vi "Restarts Monitor (FPGA).vi"() -> ()   [LabVIEW 2019]
uses:
  <vilib>/eio/EIONode/EIONode.xnode
  <vilib>/rvi/eio/common/nirviEmuTemplateMethod_errors.vi
panel:
  in  "Reset":bool
  in  "Loop Timer (uSec)":u32 caption="Count(uSec)"
  out "Actual Pump Starts":u32[](array[numeric])
  in  "Consec Samples":i32
  in  "Threshold (A)":sgl
  out "Currents (A)":sgl[](array[numeric])
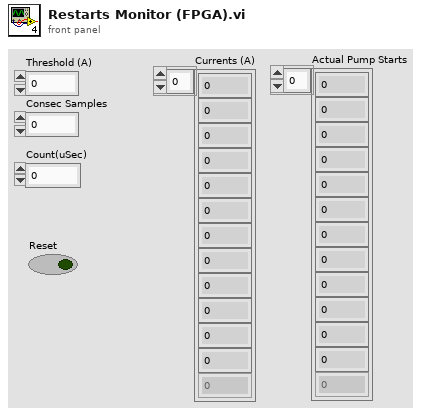
[diagram p1: front panel]
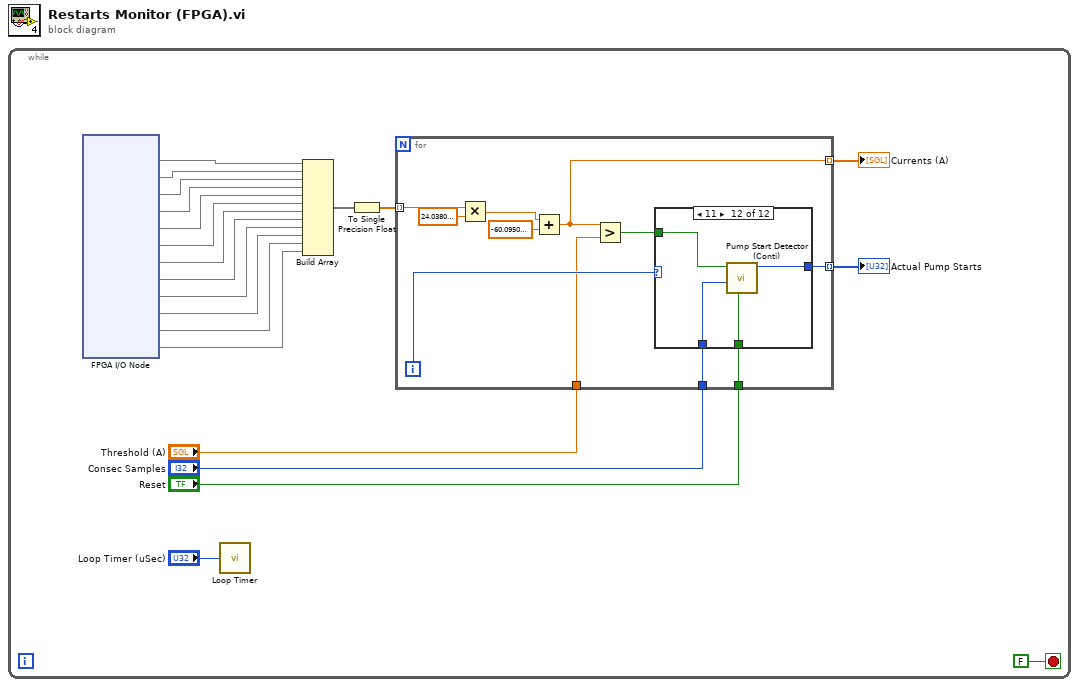
[diagram p0: block diagram]
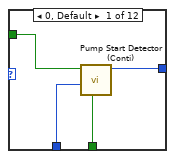
[diagram p2: hidden frame]
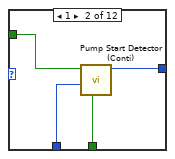
[diagram p3: hidden frame]
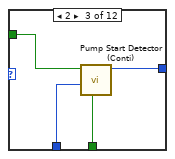
[diagram p4: hidden frame]
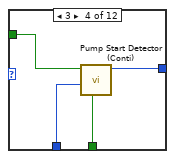
[diagram p5: hidden frame]
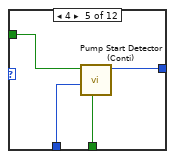
[diagram p6: hidden frame]
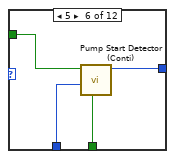
[diagram p7: hidden frame]
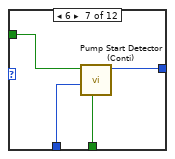
[diagram p8: hidden frame]
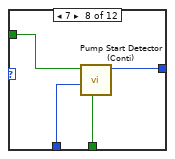
[diagram p9: hidden frame]
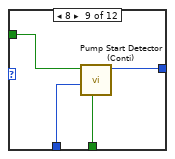
[diagram p10: hidden frame]
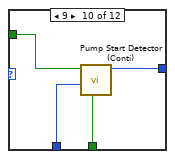
[diagram p11: hidden frame]
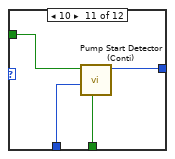
[diagram p12: hidden frame]
diagram:
  n1 = while {
    stop <- FALSE stop-if-true
    n2 = xnode "FPGA I/O Node"() -> ("AI0"=w2, "AI1"=w21, "AI2"=w20, "AI3"=w19, "AI4"=w18, "AI5"=w17, "AI6"=w16, "AI7"=w15, "AI8"=w14, "AI9"=w13, "AI10"=w12, "AI11"=w11)  [unwired: 12 in, 12 out]
    n3 = call "Loop Timer"("Count(uSec)"="Loop Timer (uSec)") -> ()  [unwired: 1 out]
    n4 = Build Array(w2, w21, w20, w19, w18, w17, w16, w15, w14, w13, w12, w11) -> (w10:void[])
    n5 = To Single Precision Float(number=w10) -> (single precision float=w9:sgl[])
    n6 = for {
      tunnel: w9 -> [w32] mode=indexing
      tunnel: [w25] -> w8 mode=indexing
      tunnel: "Consec Samples" -> [w27]
      tunnel: [w26] -> w5 mode=indexing
      tunnel: "Threshold (A)" -> [w24]
      tunnel: "Reset" -> [w22]
      i -> [w28]
      n7 = Multiply(x=w32, y=sgl 24.038) -> (x*y=w29:sgl)
      n8 = Add(x=w29, y=sgl -60.095) -> (x+y=w25:sgl)
      n9 = Greater?(x=w25, y=w24) -> (0:w23:bool)
      n10 = case shown="11" w28 {
        tunnel: w23 -> [w36 w40 w44 w48 w52 w56 w60 w64 w68 w72 w76 w78]
        tunnel: w27 -> [w35 w39 w43 w47 w51 w55 w59 w63 w67 w71 w75 w80]
        tunnel: [w34 w38 w42 w46 w50 w54 w58 w62 w66 w70 w74 w79] -> w26
        tunnel: w22 -> [w33 w37 w41 w45 w49 w53 w57 w61 w65 w69 w73 w77]
        frame 0, Default {
          n11 = call "Pump Start Detector (Conti).vi"("Reset"=w33, "Consec Samples"=w35, "Crossing?"=w36) -> ("Restarts"=w34:u32)  [unwired: 8 in]
        }
        frame 1 {
          n12 = call "Pump Start Detector (Conti).vi"("Reset"=w37, "Consec Samples"=w39, "Crossing?"=w40) -> ("Restarts"=w38:u32)  [unwired: 8 in]
        }
        frame 2 {
          n13 = call "Pump Start Detector (Conti).vi"("Reset"=w41, "Consec Samples"=w43, "Crossing?"=w44) -> ("Restarts"=w42:u32)  [unwired: 8 in]
        }
        frame 3 {
          n14 = call "Pump Start Detector (Conti).vi"("Reset"=w45, "Consec Samples"=w47, "Crossing?"=w48) -> ("Restarts"=w46:u32)  [unwired: 8 in]
        }
        frame 4 {
          n15 = call "Pump Start Detector (Conti).vi"("Reset"=w49, "Consec Samples"=w51, "Crossing?"=w52) -> ("Restarts"=w50:u32)  [unwired: 8 in]
        }
        frame 5 {
          n16 = call "Pump Start Detector (Conti).vi"("Reset"=w53, "Consec Samples"=w55, "Crossing?"=w56) -> ("Restarts"=w54:u32)  [unwired: 8 in]
        }
        frame 6 {
          n17 = call "Pump Start Detector (Conti).vi"("Reset"=w57, "Consec Samples"=w59, "Crossing?"=w60) -> ("Restarts"=w58:u32)  [unwired: 8 in]
        }
        frame 7 {
          n18 = call "Pump Start Detector (Conti).vi"("Reset"=w61, "Consec Samples"=w63, "Crossing?"=w64) -> ("Restarts"=w62:u32)  [unwired: 8 in]
        }
        frame 8 {
          n19 = call "Pump Start Detector (Conti).vi"("Reset"=w65, "Consec Samples"=w67, "Crossing?"=w68) -> ("Restarts"=w66:u32)  [unwired: 8 in]
        }
        frame 9 {
          n20 = call "Pump Start Detector (Conti).vi"("Reset"=w69, "Consec Samples"=w71, "Crossing?"=w72) -> ("Restarts"=w70:u32)  [unwired: 8 in]
        }
        frame 10 {
          n21 = call "Pump Start Detector (Conti).vi"("Reset"=w73, "Consec Samples"=w75, "Crossing?"=w76) -> ("Restarts"=w74:u32)  [unwired: 8 in]
        }
        frame 11 {
          n22 = call "Pump Start Detector (Conti).vi"("Reset"=w77, "Consec Samples"=w80, "Crossing?"=w78) -> ("Restarts"=w79:u32)  [unwired: 8 in]
        }
      }
    }
    "Currents (A)" <- w8
    "Actual Pump Starts" <- w5
  }
